vi "Write Length Z.vi"(8 "error in (no error)":errorcluster, 10 "Length Z":sgl=1.0, 11 "ODESimulator_LinearConveyor in":refnum<class "ODESimulator_LinearConveyor.lvclass">) -> (0 "error out":errorcluster, 3 "ODESimulator_LinearConveyor out":refnum<class "ODESimulator_LinearConveyor.lvclass">)   [LabVIEW 2017, in "NI_Robotics_Simulator.lvlib" / "ODESimulator_LinearConveyor.lvclass"]
uses:
  <vilib>/robotics/Simulator/Robot Factory/Conveyor/Linear/ODESimulator_LinearConveyor.lvclass
  <vilib>/robotics/Simulator/Robot Factory/Conveyor/Linear/ODESimulator_LinearConveyor.lvclass/ODESimulator_LinearConveyor.ctl
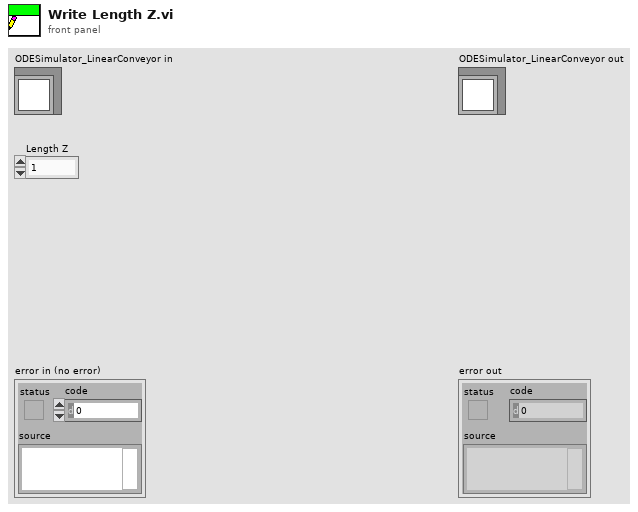
[diagram p1: front panel]
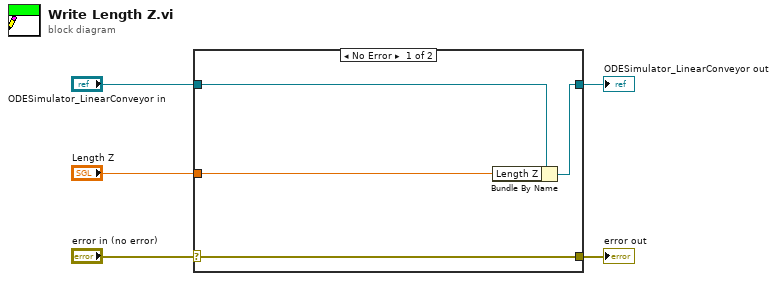
[diagram p0: block diagram]
diagram:
  n1 = case shown="No Error" "error in (no error)" {
    selector: "error in (no error)" -> [w9 w10]
    tunnel: [w9 w10] -> w4
    tunnel: [w7 w11] -> w2
    tunnel: "ODESimulator_LinearConveyor in" -> [w8 w11]
    tunnel: "Length Z" -> [w6 _]
    frame No Error {
      n2 = Bundle By Name(cluster=w8, "Length Z"=w6) -> (w7:refnum<class "ODESimulator_LinearConveyor.lvclass">)
    }
    frame Error {
    }
  }
  "error out" <- w4
  "ODESimulator_LinearConveyor out" <- w2
